vi "NetworkScan.vi"() -> ()   [LabVIEW 2013]
uses:
  Global 1.vi
panel:
  out "Freq":dbl[](array[numeric])
  out "R":dbl[](array[numeric])
  out "X":dbl[](array[numeric])
  out "Z":dbl[](array[numeric])
  out "rho":dbl[](array[numeric])
  out "X/R":dbl[](array[numeric])
  out "Smith Chart":picture
  out "Handle":u32
  out "Device Description":string="DLP-IO20"
  in  "Device Index":u32
  in  "Phase adjust":bool
  in  "Fstep":dbl=5.0 format="%#_13g"
  in  "Fmin":dbl=50.0 format="%#_13g"
  in  "Fmax (MHz)":dbl=300.0 format="%#_13g"
  out "Reflected Angle (deg)":cluster{"Fmin":dbl, "Fstep":dbl, dbl[]}(graph)
  out "Reflected Power (dBc)":cluster{"Fmin":dbl, "Fstep":dbl, dbl[]}(graph)
  # "Network Analyzer"
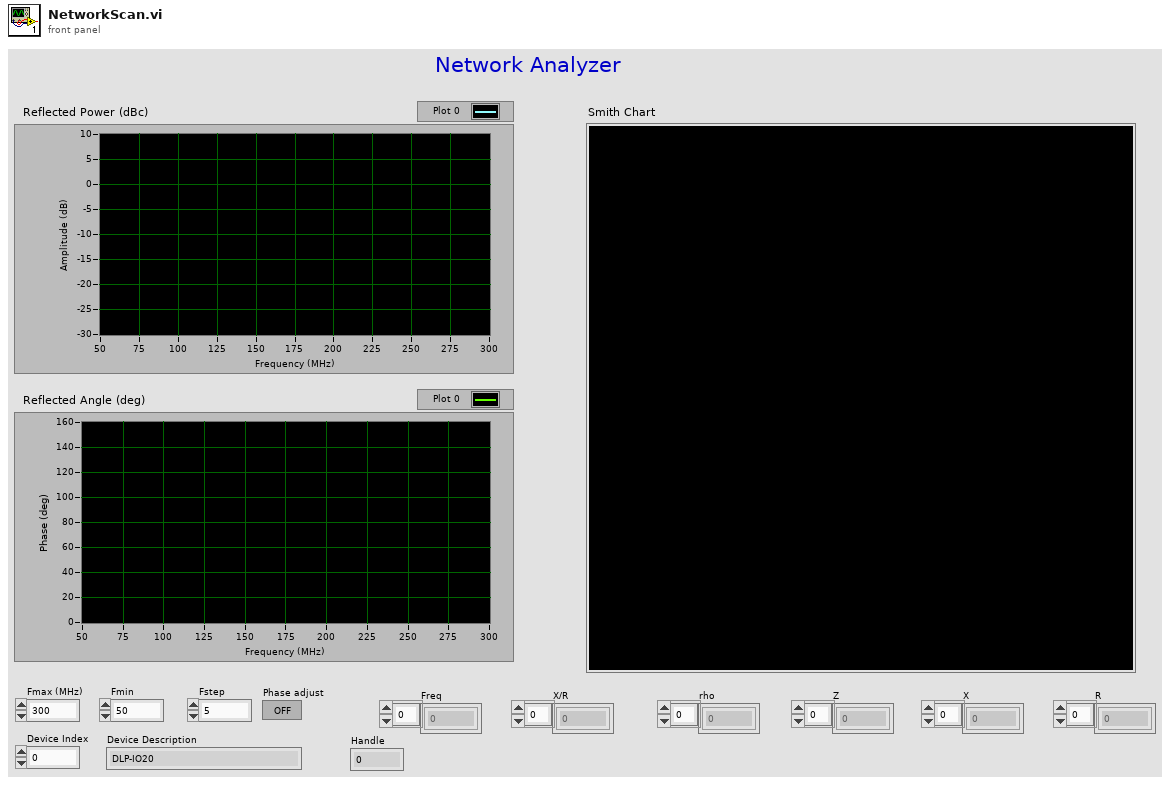
[diagram p1: front panel]
types:
  T1 = typedef "LVBoundsTypeDef.ctl" = cluster{"Width":u32, "Height":u32}
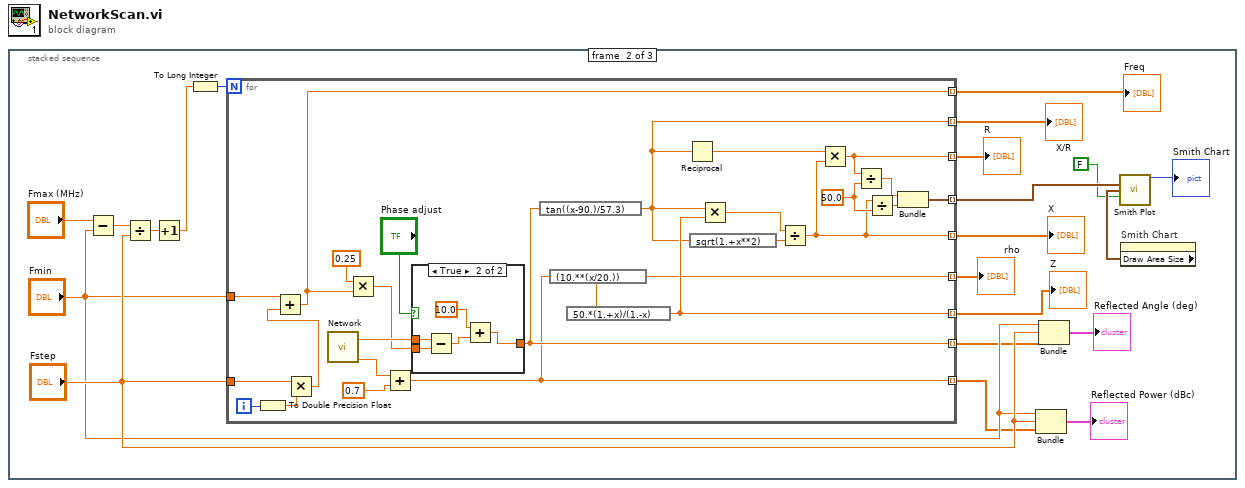
[diagram p0: block diagram]
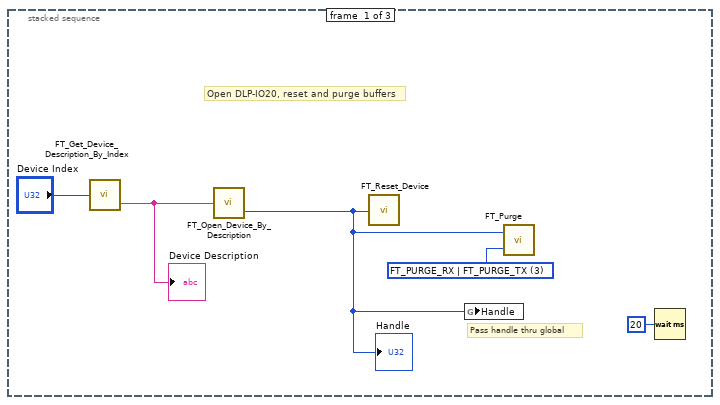
[diagram p2: hidden frame]
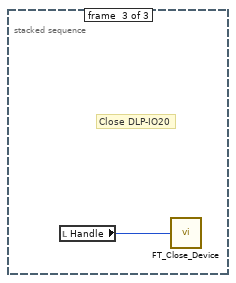
[diagram p4: hidden frame]
diagram:
  n1 = stacked-sequence {
    frame #0 {
      w3 = u32 3 items=["FT_PURGE_RX"=1, "FT_PURGE_TX"=2, "FT_PURGE_RX | FT_PURGE_TX"=3] ("Purge Flags")
      # "Pass handle thru global"
      # "Open DLP-IO20, reset and purge buffers"
      n2 = call "FT_Get_Device_Description_By_Index.vi"("Device Index"="Device Index") -> ("Device Description"=w4:string)  [unwired: 1 out]
      "Device Description" <- w4
      n3 = call "FT_Open_Device_By_Description.vi"("Device Description"=w4) -> ("Handle"=w1:u32)  [unwired: 1 out]
      "Handle" <- w1
      n4 = call "FT_Reset_Device.vi"("Handle"=w1) -> ()  [unwired: 1 out]
      n5 = global write "Global 1.vi" "Handle"(w1) -> ()
      n6 = call "FT_Purge.vi"("Purge Flags"=w3, "Handle"=w1) -> ()  [unwired: 1 out]
      n7 = Wait (ms)(milliseconds to wait=u32 20) -> ()  [unwired: 1 out]
    }
    frame #1 {
      n8 = Subtract(x="Fmax (MHz)", y="Fmin") -> (x-y=w23:dbl)
      n9 = Divide(x=w23, y="Fstep") -> (x/y=w20:dbl)
      n10 = Increment(x=w20) -> (x+1=w21:dbl)
      n11 = To Long Integer(number=w21) -> (32bit integer=w22:i32)
      n12 = for {
        N: w22 -> [_]
        tunnel: [w37] -> w16 mode=indexing
        tunnel: [w38] -> w17 mode=indexing
        tunnel: "Fmin" -> [w47]
        tunnel: "Fstep" -> [w49]
        tunnel: [w36] -> w15 mode=indexing
        tunnel: [w35] -> w14 mode=indexing
        tunnel: [w34] -> w13 mode=indexing
        tunnel: [w28] -> w12 mode=indexing
        tunnel: [w32] -> w11 mode=indexing
        tunnel: [w33] -> w8 mode=indexing
        tunnel: [w27] -> w6 mode=indexing
        i -> [w50]
        w29 = 50.0
        n13 = To Double Precision Float(number=w50) -> (double precision float=w48:dbl)
        n14 = Multiply(x=w49, y=w48) -> (x*y=w46:dbl)
        n15 = Add(x=w47, y=w46) -> (x+y=w27:dbl)
        n16 = call "Network.vi"() -> ("dB refl"=w51:dbl, "deg refl"=w44:dbl)  [unwired: 2 out]
        n17 = Multiply(x=0.25, y=w27) -> (x*y=w43:dbl)
        n18 = Add(x=w51, y=0.7) -> (x+y=w37:dbl)
        n19 = case shown="True" "Phase adjust" {
          tunnel: w44 -> [w53 w58]
          tunnel: w43 -> [_ w57]
          tunnel: [w53 w55] -> w38
          frame False {
          }
          frame True {
            n20 = Subtract(x=w58, y=w57) -> (x-y=w56:dbl)
            n21 = Add(x=10.0, y=w56) -> (x+y=w55:dbl)
          }
        }
        n22 = expression code="tan((x-90.)/57.3)"(w38) -> (w34:dbl)
        n23 = expression code="(10.**(x/20.))"(w37) -> (w35:dbl)
        n24 = expression code="50.*(1.+x)/(1.-x)"(w35) -> (w36:dbl)
        n25 = Reciprocal(x=w34) -> (1/x=w39:dbl)
        n26 = expression code="sqrt(1.+x**2)"(w34) -> (w40:dbl)
        n27 = Multiply(x=w34, y=w36) -> (x*y=w41:dbl)
        n28 = Divide(x=w41, y=w40) -> (x/y=w28:dbl)
        n29 = Multiply(x=w39, y=w28) -> (x*y=w32:dbl)
        n30 = Divide(x=w32, y=w29) -> (x/y=w31:dbl)
        n31 = Divide(x=w28, y=w29) -> (x/y=w30:dbl)
        n32 = Bundle(w31, w30) -> (w33:cluster{dbl, dbl})  [unwired: 1 in]
      }
      "Z" <- w15
      "X" <- w12
      "R" <- w11
      "X/R" <- w13
      "rho" <- w14
      "Freq" <- w6
      n33 = Bundle("Fmin"="Fmin", "Fstep"="Fstep", w16) -> (→"Reflected Power (dBc)":cluster{"Fmin":dbl, "Fstep":dbl, dbl[]})  [unwired: 1 in]
      n34 = Bundle("Fmin"="Fmin", "Fstep"="Fstep", w17) -> (→"Reflected Angle (deg)":cluster{"Fmin":dbl, "Fstep":dbl, dbl[]})  [unwired: 1 in]
      n35 = property on="Smith Chart" class="Pict"() -> ("Draw Area Size"=w9:T1)  [unwired: 2 in, 2 out]
      n36 = call <vilib>:"Smith Plot.vi"("smith plot"=w8, "dimensions (w,h)"=w9, "dimensions incl scales? (T)"=FALSE) -> ("new picture"=→"Smith Chart":picture)  [unwired: 12 in]
    }
    frame #2 {
      # "Close DLP-IO20"
      n37 = local read "Handle"() -> (w59:u32)
      n38 = call "FT_Close_Device.vi"("Handle"=w59) -> ()  [unwired: 1 out]
    }
  }
